vi "FPGA_Throughput.vi"() -> ()   [LabVIEW 2010]
uses:
  <vilib>/Platform/TimedLoop/XDataNode/XDataNode.xnode
  <vilib>/Platform/TimedLoop/XDataNode/timing_clust.ctl
  <vilib>/Platform/TimedLoop/XDataNode/nitl_modes.ctl
  <vilib>/Platform/TimedLoop/XDataNode/wakeup.ctl
  FPGAWrapperRK110512Fiber/FPGA_Typedefs/channels_array.ctl
  FPGAWrapperRK110512Fiber/FPGA_Typedefs/pixel_to_host_enum.ctl
  <vilib>/Platform/TimedLoop/XDataNode/XDNodeRunTimeDep.lvlib
panel:
  in  "Cycles":u16
  in  "Generate":bool
  in  "Quit":bool
  out "FIFO overflow out":bool
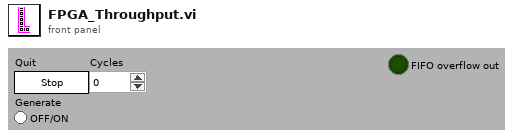
[diagram p1: front panel]
types:
  T1 = typedef "XDNodeRunTimeDep.lvlib/timing_clust.ctl" = cluster{"Expected End [f-1]":u64, "Actual End [f-1]":u64, "Finished Late? [f-1]":bool, "Expected End [i-1]":u64, "Actual End [i-1]":u64, "Finished Late? [i-1]":bool, "Expected Start [i]":u64, "Actual Start [i]":u64, "Expected Start [f]":u64, "Actual Start [f]":u64, "Source Name":string, "Structure Name":string, "Period":i64, "Deadline":i64, "Offset":i64, "Start":i64, "Priority":i32, "Timeout":i32, "Mode":T2, "Wakeup Reason":T3, "Error":errorcluster, "Source Type":string, "Secondary Source Type":string, "Global End Time":u64, "Global Start Time":u64, "Frame Duration":u64, "Iteration Duration":u64, "Assigned CPU":i32, "I/O Scan Engine Mode":u32}
  T2 = typedef "XDNodeRunTimeDep.lvlib/nitl_modes.ctl" = enum32{"No Change", "Process missed periods, maintain original phase", "Discard missed periods, maintain original phase", "Process missed periods, ignore original phase", "Discard missed periods, ignore original phase"}
  T3 = typedef "XDNodeRunTimeDep.lvlib/wakeup.ctl" = enum32{"Normal", "Aborted", "Asynchronous wakeup", "Timing source error", "Timed loop error", "Timeout"}
  T4 = typedef "channels_array.ctl" = cluster{"channel 0":u32, "channel 1":u32, "channel 2":u32, "channel 3":u32}
  T5 = typedef "pixel_to_host_enum.ctl" = enum16{"four-channel mode", "two-channel mode"}
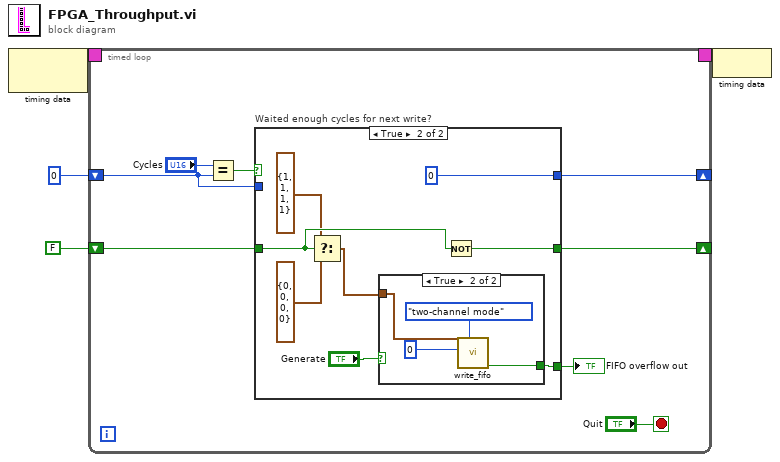
[diagram p0: block diagram]
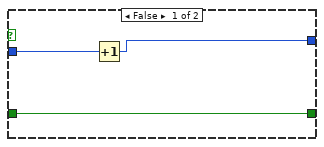
[diagram p2: hidden frame]
diagram:
  n1 = node-c288() -> (w4:T1)  [unwired: 1 in]
  n2 = timed-loop {
    timing: w4 -> [_]
    timing-out: [_] -> w3
    shift-right: [w8] -> _
    shift-left: u16 0 -> [w9]
    shift-right: [w5] -> _
    shift-left: FALSE -> [w6]
    stop <- "Quit" stop-if-true
    n3 = Equal?(x="Cycles", y=w9) -> (x = y?=w7:bool)
    n4 = case "Waited enough cycles for next write?" shown="True" w7 {
      tunnel: [_ w23] -> w12
      tunnel: w9 -> [w15 _]
      tunnel: [w14 u16 0] -> w8
      tunnel: w6 -> [w13 w18]
      tunnel: [w13 w19] -> w5
      frame False {
        n5 = Increment(x=w15) -> (x+1=w14:u16)
      }
      frame True {
        n6 = Select(t=T4 {"channel 0"=1, "channel 1"=1, "channel 2"=1, "channel 3"=1} ("values to be written"), s=w18, f=T4 {"channel 0"=0, "channel 1"=0, "channel 2"=0, "channel 3"=0} ("values to be written")) -> (s? t:f=w20:T4)
        n7 = case shown="True" "Generate" {
          tunnel: [_ w27] -> w23
          tunnel: w20 -> [_ w24]
          frame False {
          }
          frame True {
            n8 = call "write_fifo.vi"("pixel-to-host\n mode"=pixel_to_host_enum."two-channel mode" ("pixel-to-host\n mode"), "block index in"=0 ("maximum bit depth"), "values to be written"=w24) -> ("FIFO overflow out"=w27:bool)  [unwired: 6 in, 2 out]
          }
        }
        n9 = Not(x=w18) -> (.not. x?=w19:bool)
      }
    }
    "FIFO overflow out" <- w12
  }
  n10 = node-c288(w3) -> ()
